vi "Alex Fails.vi"() -> ()   [LabVIEW 2014]
doc: "This VI is called when autonomous begins, and will automatically be terminated when autonomous ends. You can carry out timed or sensor driven robot movement independently without needing to return to the caller."
uses:
  Robot/Auto/Autonomous Modes.ctl
  Robot/Main/Elevator/Elevator States.ctl
  Robot/Main/Arms/Arm clapper state.ctl
  <vilib>/Rock Robotics/Network Tables/SD Read Number.vi
panel:
  in  "Forward Speed 2":dbl=0.8
  in  "Forward Speed":dbl=0.55 format="%#_13g"
  in  "Distance (in)":dbl=108.0
  in  "Turn Left Distance (m)":dbl=108.0 format="%#_13g"
  in  "Turn Left Speed":dbl=0.5
  in  "Turn Right Speed":dbl=0.5
  in  "Turn Right Distance (m)":dbl=108.0 format="%#_13g"
  in  "Move Speed":dbl=0.5 format="%#_13g"
  in  "Move Time (s)":dbl=2.5 format="%#_13g"
  # "THREE TOTE"
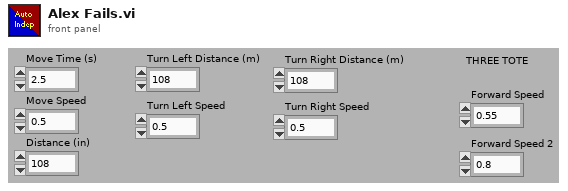
[diagram p1: front panel]
types:
  T1 = typedef "Autonomous Modes.ctl" = enum16{"3 Tote", "Turn Left, Drive to Auto", "Turn Right, Drive to Auto", "1 Bin", "Move To Auto Zone", "Do Nothing"}
  T2 = typedef "Auto Notifiers.ctl" = cluster{"Auto to Clap":refnum<notifier>, "Clap to Auto":refnum<notifier>, "Auto to Angle":refnum<notifier>, "Angle to Auto":refnum<notifier>, "Auto to Roller":refnum<notifier>, "Drive Distance Speed":refnum<notifier>, "Drive Distance Distance":refnum<notifier>, "Auto Done?":refnum<notifier>, "Keep Straight?":refnum<notifier>, "Turn 90?":refnum<notifier>}
  T3 = typedef "Auto Refs.ctl" = cluster{"Ultrasonic Forward":T4, "Ultrasonic Back":T4, "Strafe Motor":T8, "Drive Motors":T17, "Gyro":T18}
  T4 = typedef "WPI_SonarMB1010AnalogDeviceRef.ctl" = cluster{"AIDeviceRef":T5, "Scaling factor (V/in)":dbl, "Average Bits":u8}
  T5 = typedef "WPI_AnalogChannelDevRef.ctl" = cluster{"DevStatus":errorcluster, "Controller":T6, "Analog Channel":T7}
  T6 = typedef "FPGA_TypedefAnalogModule.ctl" = enum16{"Controller 1"}
  T7 = typedef "FPGA_AIChannel.ctl" = enum8{"AI 0", "AI 1", "AI 2", "AI 3", "AI MXP 0", "AI MXP 1", "AI MXP 2", "AI MXP 3", "Invalid"}
  T8 = typedef "WPI_MotorControlDeviceRef.ctl" = cluster{"DeviceStatus":errorcluster, "Type":T9, "PWM":cluster{"Controller":T10, "PWM Channel":T11, "DeadBand":T12}, "CAN":cluster{"Device Number":u8, "Control Mode":T13, "Semaphore":T14, "Max Vout":dbl, "TalonSRX Control Mode":T15}, "Invert":bool, "TransformRef":T16, "InvTransformRef":T16}
  T9 = typedef "WPI_MotorControlType.ctl" = enum16{"PWM", "CAN", "CANTalonSRX"}
  T10 = typedef "FPGA_TypedefDigitalModule.ctl" = enum16{"Controller 1"}
  T11 = typedef "FPGA_DIOPWMChannel.ctl" = enum8{"PWM 0", "PWM 1", "PWM 2", "PWM 3", "PWM 4", "PWM 5", "PWM 6", "PWM 7", "PWM 8", "PWM 9", "PWM MXP 0", "PWM MXP 1", "PWM MXP 2", "PWM MXP 3", "PWM MXP 4", "PWM MXP 5", "PWM MXP 6", "PWM MXP 7", "PWM MXP 8", "PWM MXP 9", "Invalid"}
  T12 = typedef "WPI_PWMDeadband.ctl" = cluster{"Name":string, "maxPositivePwm":i32, "minPositivePwm":i32, "centerPwm":i32, "maxNegativePwm":i32, "minNegativePwm":i32, "angularRange":u16}
  T13 = typedef "WPI_CANJaguar_ControlMode.ctl" = enum8{"Percent VBus", "Current", "Speed", "Position", "Voltage"}
  T14 = typedef "Semaphore RefNum" = refnum<k1>
  T15 = typedef "WPI_CANTalonSRX_APIControlMode.ctl" = enum8{"Percent VBus", "Speed", "Position", "Slave", "Unchanged / Invalid"}
  T16 = typedef "WPI_PWMTransform_ConPane.ctl" = refnum<vi>
  T17 = typedef "WPI_RobotDriveDevRef.ctl" = cluster{"DevStatus":errorcluster, "Motors[]":T8[], "Square Inputs":bool, "Max Output":dbl}
  T18 = typedef "WPI_GyroDevRef.ctl" = cluster{"DevStatus":errorcluster, "Analog Module":T6, "Analog Channel":T7, "Offset":dbl, "Gain (VoltsPerDegree/Second)":dbl}
  T19 = typedef "Arm clapper state.ctl" = enum16{"In", "Tote Closed", "Bin Closed", "Straight", "Open"}
  T20 = typedef "Elevator States.ctl" = enum16{"Ground", "Tote 1", "Tote 2", "Tote 3", "Tote 4", "Tote 5", "Tote 6"}
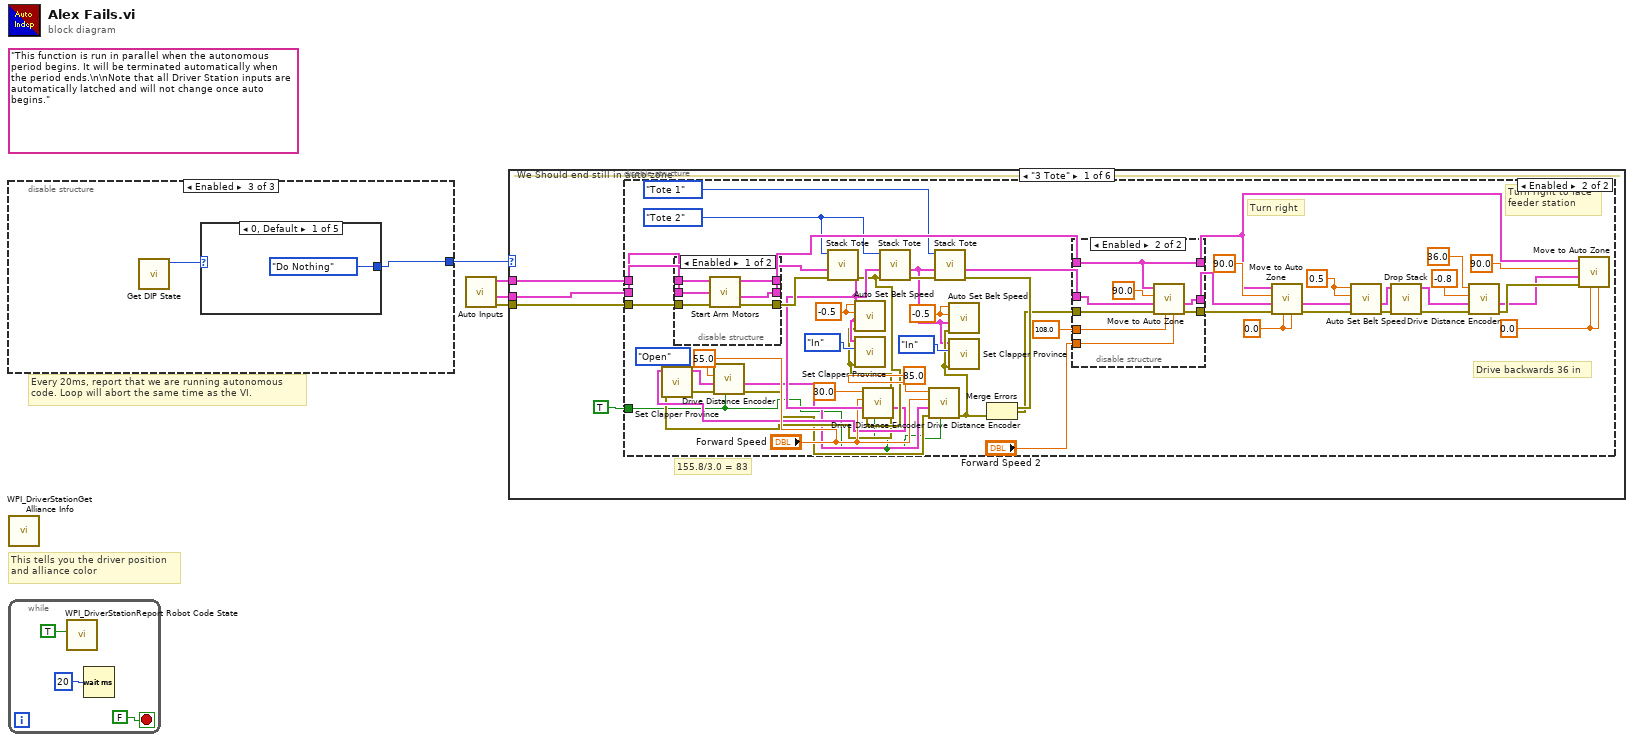
[diagram p0: block diagram]
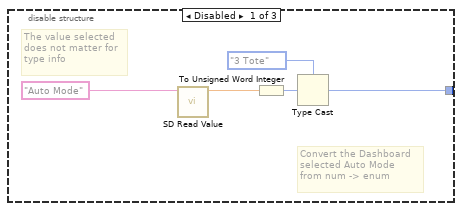
[diagram p2: hidden frame]
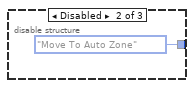
[diagram p3: hidden frame]
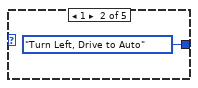
[diagram p4: hidden frame]
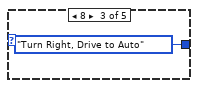
[diagram p5: hidden frame]
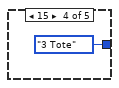
[diagram p6: hidden frame]
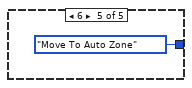
[diagram p7: hidden frame]
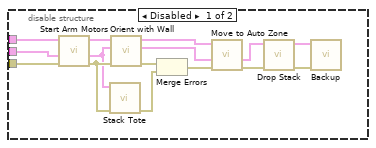
[diagram p8: hidden frame]
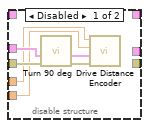
[diagram p10: hidden frame]
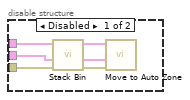
[diagram p12: hidden frame]
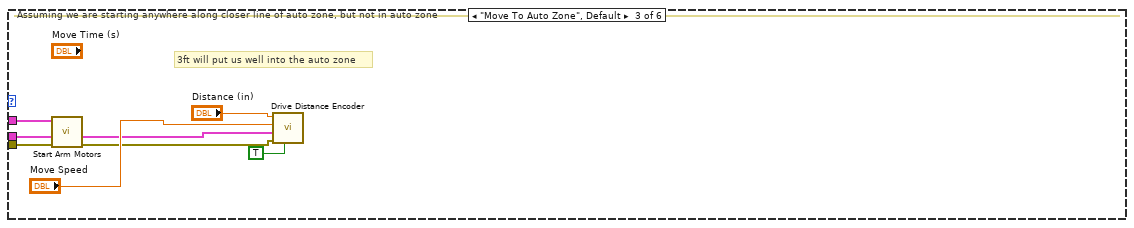
[diagram p13: hidden frame]
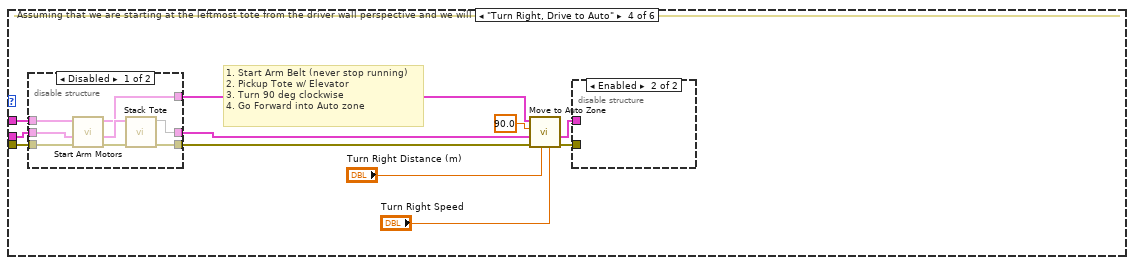
[diagram p14: hidden frame]
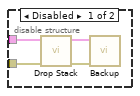
[diagram p15: hidden frame]
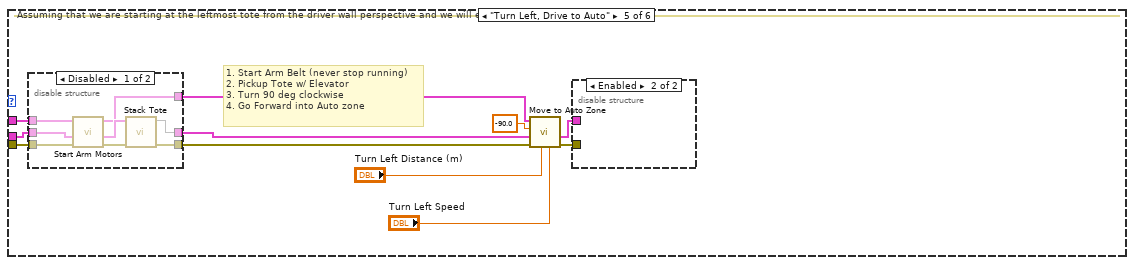
[diagram p17: hidden frame]
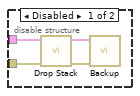
[diagram p18: hidden frame]
diagram:
  (unwired) "This function is run in parallel when the autonomous period begins. It will be terminated automatically when the period ends.\n\nNote that all Driver Station inputs are automatically latched and will not change once auto begins."
  # "Every 20ms, report that we are running autonomous\ncode. Loop will abort the same time as the VI."
  # "This tells you the driver position\nand alliance color"
  n1 = disable-structure shown="Enabled" {
    disable-tunnel: [w5 Autonomous_Modes."Move To Auto Zone" ("Auto Mode") w11] -> w1
    frame Disabled {
      # "The value selected\ndoes not matter for\ntype info"
      # "Convert the Dashboard\nselected Auto Mode\nfrom num -> enum"
      n2 = call-poly <vilib>:"SD Read Value.vi"("Name"="Auto Mode") -> ("Numeric"=w9:dbl)  [unwired: 8 in, 2 out]
      n3 = To Unsigned Word Integer(number=w9) -> (unsigned 16bit integer=w8:u16)
      n4 = Type Cast(type=Autonomous_Modes."3 Tote" ("Auto Mode"), x=w8) -> (*(type *) &x=w5:T1)
    }
    frame Disabled {
    }
    frame Enabled {
      n5 = call "Get DIP State.vi"() -> ("DIP State"=w12:u32)  [unwired: 10 in, 1 out]
      n6 = case shown="0, Default" w12 {
        tunnel: [Autonomous_Modes."Do Nothing" ("Auto Mode") Autonomous_Modes."Turn Left, Drive to Auto" ("Auto Mode") Autonomous_Modes."Turn Right, Drive to Auto" ("Auto Mode") Autonomous_Modes."3 Tote" ("Auto Mode") Autonomous_Modes."Move To Auto Zone" ("Auto Mode")] -> w11
        frame 0, Default {
        }
        frame 1 {
        }
        frame 8 {
        }
        frame 15 {
        }
        frame 6 {
        }
      }
    }
  }
  n7 = call <vilib>:"WPI_DriverStationGet Alliance Info.vi"() -> ()  [unwired: 12 out]
  n8 = while {
    stop <- FALSE stop-if-true
    n9 = call <vilib>:"WPI_DriverStationReport Robot Code State.vi"("Autonomous"=TRUE) -> ()  [unwired: 10 in, 1 out]
    n10 = Wait (ms)(milliseconds to wait=u32 20) -> ()  [unwired: 1 out]
  }
  n11 = call "Auto Inputs.vi"() -> ("error out"=w2:errorcluster, "Auto Notifiers Out"=w3:T2, "Auto Refs"=w4:T3)  [unwired: 9 in]
  n12 = case shown="\"3 Tote\"" w1 {
    tunnel: w4 -> [w22 w117 w126 w136 w162 _]
    tunnel: w3 -> [w24 w116 w128 w140 w166 _]
    tunnel: w2 -> [w23 w115 w130 w139 w165 _]
    frame "3 Tote" {
      # "155.8/3.0 = 83"
      # "We Should end still in auto zone"
      n13 = disable-structure shown="Enabled" {
        disable-tunnel: w24 -> [w32 w90]
        disable-tunnel: w23 -> [w31 w91]
        disable-tunnel: w22 -> [w25 w89]
        disable-tunnel: TRUE -> [_ w40]
        frame Disabled {
          n14 = call "Start Arm Motors.vi"("error in"=w31, "Auto Notifiers In"=w32, "Auto Refs"=w25) -> ("error out"=w37:errorcluster, "Auto Notifiers Out"=w34:T2, "Auto Refs"=w36:T3)  [unwired: 6 in]
          n15 = call "Stack Tote.vi"("error in"=w37, "End at"=w34) -> ("error out"=w38:errorcluster)  [unwired: 8 in, 1 out]
          n16 = call "Orient with Wall.vi"("error in"=w37, "Auto Notifiers In"=w34, "Auto Refs"=w36) -> ("error out"=w35:errorcluster, "Auto Notifiers Out"=w33:T2, "Auto Refs"=w26:T3)  [unwired: 6 in]
          n17 = Merge Errors(w35, w38) -> (w39:errorcluster)
          n18 = call "Move to Auto Zone.vi"("error in"=w39, "Auto Notifiers In"=w33, "Auto Refs"=w26) -> ("error out"=w29:errorcluster, "Auto Notifiers Out"=w28:T2)  [unwired: 7 in]
          n19 = call "Drop Stack.vi"("error in"=w29, "Auto Notifiers In"=w28) -> ("error out"=w30:errorcluster, "Auto Notifiers Out"=w27:T2)  [unwired: 8 in]
          n20 = call "Backup.vi"("error in"=w30, "Auto Notifiers In"=w27) -> ()  [unwired: 8 in, 2 out]
        }
        frame Enabled {
          w56 = -0.5 ("Right Belt")
          w57 = -0.5 ("Right Belt")
          w73 = Elevator_States."Tote 2" ("New State")
          w81 = 0.0 ("Distance (m)")
          w82 = 0.0 ("Distance (m)")
          w61 = 0.5
          # "Drive backwards 36 in"
          # "Turn right to face\nfeeder station"
          # "Turn right"
          n21 = disable-structure shown="Enabled" {
            disable-tunnel: w91 -> [w97 w98]
            disable-tunnel: w90 -> [w96 w100]
            disable-tunnel: w89 -> [w95 w99]
            disable-tunnel: [w94 w98] -> w77
            disable-tunnel: [w93 w100] -> w78
            disable-tunnel: [w92 w99] -> w86
            frame Enabled {
              n22 = call "Start Arm Motors.vi"("error in"=w97, "Auto Notifiers In"=w96, "Auto Refs"=w95) -> ("error out"=w94:errorcluster, "Auto Notifiers Out"=w93:T2, "Auto Refs"=w92:T3)  [unwired: 6 in]
            }
            frame Disabled {
            }
          }
          n23 = call "Stack Tote.vi"("error in"=w77, "Auto Notifiers In"=w78, "End at"=w73) -> ("error out"=w51:errorcluster, "Auto Notifiers Out"=w52:T2)  [unwired: 7 in]
          n24 = call "Drive Distance Encoder.vi"("Gyro Sync?"=w40, "error in"=w51, "Auto Notifiers In"=w52, "Speed"="Forward Speed", "Distance (in)"=30.0) -> ("error out"=w43:errorcluster, "Auto Notifiers Out"=w44:T2)  [unwired: 5 in]
          n25 = call "Set Clapper Province.vi"("error in"=w43, "Enum"=Arm_clapper_state."Open", "Auto Notifiers In"=w44) -> ("error out"=w47:errorcluster, "Auto Notifiers Out"=w48:T2)  [unwired: 7 in]
          n26 = call "Drive Distance Encoder.vi"("Gyro Sync?"=w40, "error in"=w47, "Auto Notifiers In"=w48, "Speed"="Forward Speed", "Distance (in)"=55.0) -> ("error out"=w42:errorcluster, "Auto Notifiers Out"=w41:T2)  [unwired: 5 in]
          n27 = call "Auto Set Belt Speed.vi"("error in"=w43, "Auto Notifiers In"=w52, "Right Belt"=w57, "Left Belt"=w57) -> ()  [unwired: 6 in, 2 out]
          n28 = call "Set Clapper Province.vi"("error in"=w43, "Enum"=Arm_clapper_state."In", "Auto Notifiers In"=w52) -> ()  [unwired: 7 in, 2 out]
          n29 = call "Stack Tote.vi"("error in"=w51, "Auto Notifiers In"=w52, "End at"=w73) -> ("error out"=w76:errorcluster, "Auto Notifiers Out"=w53:T2)  [unwired: 7 in]
          n30 = call "Drive Distance Encoder.vi"("Gyro Sync?"=w40, "error in"=w42, "Auto Notifiers In"=w41, "Speed"="Forward Speed", "Distance (in)"=85.0) -> ("error out"=w54:errorcluster)  [unwired: 5 in, 1 out]
          n31 = call "Stack Tote.vi"("error in"=w76, "Auto Notifiers In"=w53, "End at"=Elevator_States."Tote 1" ("New State")) -> ("error out"=w75:errorcluster, "Auto Notifiers Out"=w88:T2)  [unwired: 7 in]
          n32 = call "Auto Set Belt Speed.vi"("error in"=w54, "Auto Notifiers In"=w53, "Right Belt"=w56, "Left Belt"=w56) -> ()  [unwired: 6 in, 2 out]
          n33 = call "Set Clapper Province.vi"("error in"=w54, "Enum"=Arm_clapper_state."In", "Auto Notifiers In"=w53) -> ()  [unwired: 7 in, 2 out]
          n34 = Merge Errors(w75, w54) -> (w74:errorcluster)
          n35 = disable-structure shown="Enabled" {
            disable-tunnel: w74 -> [w106 w114]
            disable-tunnel: w88 -> [w105 w113]
            disable-tunnel: "Forward Speed 2" -> [w102 w110]
            disable-tunnel: 108.0 ("Distance (in)") -> [w101 w111]
            disable-tunnel: w86 -> [_ w107]
            disable-tunnel: [_ w109] -> w85
            disable-tunnel: [_ w108] -> w84
            disable-tunnel: [_ w107] -> w79
            frame Disabled {
              n36 = call "Turn 90 deg.vi"("error in"=w106, "Auto Notifiers In"=w105) -> ("error out"=w104:errorcluster, "Auto Notifiers Out"=w103:T2)  [unwired: 8 in]
              n37 = call "Drive Distance Encoder.vi"("error in"=w104, "Auto Notifiers In"=w103, "Speed"=w102, "Distance (in)"=w101) -> ()  [unwired: 6 in, 2 out]
            }
            frame Enabled {
              n38 = call "Move to Auto Zone.vi"("Speed"=w110, "Distance (m)"=w111, "error in"=w114, "Auto Notifiers In"=w113, "Rotation (deg)"=90.0, "Auto Refs"=w107) -> ("error out"=w109:errorcluster, "Auto Notifiers Out"=w108:T2)  [unwired: 4 in]
            }
          }
          n39 = call "Move to Auto Zone.vi"("Speed"=w82, "Distance (m)"=w82, "error in"=w85, "Auto Notifiers In"=w84, "Rotation (deg)"=90.0, "Auto Refs"=w79) -> ("error out"=w63:errorcluster, "Auto Notifiers Out"=w62:T2)  [unwired: 4 in]
          n40 = call "Auto Set Belt Speed.vi"("error in"=w63, "Auto Notifiers In"=w62, "Right Belt"=w61, "Left Belt"=w61) -> ("error out"=w65:errorcluster, "Auto Notifiers Out"=w64:T2)  [unwired: 6 in]
          n41 = call "Drop Stack.vi"("error in"=w65, "Auto Notifiers In"=w64) -> ("error out"=w67:errorcluster, "Auto Notifiers Out"=w66:T2)  [unwired: 8 in]
          n42 = call "Drive Distance Encoder.vi"("error in"=w67, "Auto Notifiers In"=w66, "Speed"=-0.8, "Distance (in)"=36.0) -> ("error out"=w69:errorcluster, "Auto Notifiers Out"=w68:T2)  [unwired: 6 in]
          n43 = call "Move to Auto Zone.vi"("Speed"=w81, "Distance (m)"=w81, "error in"=w69, "Auto Notifiers In"=w68, "Rotation (deg)"=90.0 ("Distance (in)"), "Auto Refs"=w79) -> ()  [unwired: 4 in, 2 out]
        }
      }
    }
    frame "1 Bin" {
      # "1. Pick Up Bin w/ Elevator\n2. Turn 90 deg counterclockwise\n3. Go forward into auto zone\n4. DO NOT drop bin"
      # "Assuming we are starting on top of the leftmost bin from the driver wall perspective and we will end in auto zone"
      n44 = disable-structure shown="Enabled" {
        disable-tunnel: w117 -> [w121 _]
        disable-tunnel: w116 -> [w120 _]
        disable-tunnel: w115 -> [w118 _]
        frame Disabled {
          n45 = call "Stack Bin.vi"("error in"=w118, "Auto Notifiers In"=w120, "Auto Refs"=w121) -> ("error out"=w123:errorcluster, "Auto Notifiers Out"=w119:T2, "Auto Refs"=w122:T3)  [unwired: 6 in]
          n46 = call "Move to Auto Zone.vi"("error in"=w123, "Auto Notifiers In"=w119, "Auto Refs"=w122) -> ()  [unwired: 7 in, 2 out]
        }
        frame Enabled {
        }
      }
    }
    frame "Move To Auto Zone", Default {
      # "3ft will put us well into the auto zone"
      # "Assuming we are starting anywhere along closer line of auto zone, but not in auto zone"
      n47 = call "Start Arm Motors.vi"("error in"=w130, "Auto Notifiers In"=w128, "Auto Refs"=w126) -> ("error out"=w129:errorcluster, "Auto Notifiers Out"=w127:T2)  [unwired: 6 in, 1 out]
      n48 = call "Drive Distance Encoder.vi"("Gyro Sync?"=TRUE, "error in"=w129, "Auto Notifiers In"=w127, "Speed"="Move Speed", "Distance (in)"="Distance (in)") -> ()  [unwired: 5 in, 2 out]
    }
    frame "Turn Right, Drive to Auto" {
      # "1. Start Arm Belt (never stop running)\n2. Pickup Tote w/ Elevator\n3. Turn 90 deg clockwise\n4. Go Forward into Auto zone"
      # "Assuming that we are starting at the leftmost tote from the driver wall perspective and we will end in auto zone"
      n49 = disable-structure shown="Disabled" {
        disable-tunnel: [w154 w155] -> w141
        disable-tunnel: w140 -> [w152 w156]
        disable-tunnel: w139 -> [w151 w155]
        disable-tunnel: [w149 w156] -> w138
        disable-tunnel: w136 -> [w148 w157]
        disable-tunnel: [w147 w157] -> w135
        frame Disabled {
          n50 = call "Start Arm Motors.vi"("error in"=w151, "Auto Notifiers In"=w152, "Auto Refs"=w148) -> ("error out"=w153:errorcluster, "Auto Notifiers Out"=w150:T2, "Auto Refs"=w147:T3)  [unwired: 6 in]
          n51 = call "Stack Tote.vi"("error in"=w153, "End at"=w150) -> ("error out"=w154:errorcluster, 3:w149)  [unwired: 7 in, 1 out]
        }
        frame Enabled {
        }
      }
      n52 = call "Move to Auto Zone.vi"("Speed"="Turn Right Speed", "Distance (m)"="Turn Right Distance (m)", "error in"=w141, "Auto Notifiers In"=w138, "Rotation (deg)"=90.0, "Auto Refs"=w135) -> ("error out"=w142:errorcluster, "Auto Notifiers Out"=w137:T2)  [unwired: 4 in]
      n53 = disable-structure shown="Enabled" {
        disable-tunnel: w142 -> [w145 _]
        disable-tunnel: w137 -> [w144 _]
        frame Disabled {
          n54 = call "Drop Stack.vi"("error in"=w145, "Auto Notifiers In"=w144) -> ("error out"=w146:errorcluster, "Auto Notifiers Out"=w143:T2)  [unwired: 8 in]
          n55 = call "Backup.vi"("error in"=w146, "Auto Notifiers In"=w143) -> ()  [unwired: 8 in, 2 out]
        }
        frame Enabled {
        }
      }
    }
    frame "Turn Left, Drive to Auto" {
      # "1. Start Arm Belt (never stop running)\n2. Pickup Tote w/ Elevator\n3. Turn 90 deg clockwise\n4. Go Forward into Auto zone"
      # "Assuming that we are starting at the leftmost tote from the driver wall perspective and we will end in auto zone"
      n56 = disable-structure shown="Disabled" {
        disable-tunnel: [w180 w181] -> w167
        disable-tunnel: w166 -> [w178 w182]
        disable-tunnel: w165 -> [w177 w181]
        disable-tunnel: [w175 w182] -> w164
        disable-tunnel: w162 -> [w174 w183]
        disable-tunnel: [w173 w183] -> w161
        frame Disabled {
          n57 = call "Start Arm Motors.vi"("error in"=w177, "Auto Notifiers In"=w178, "Auto Refs"=w174) -> ("error out"=w179:errorcluster, "Auto Notifiers Out"=w176:T2, "Auto Refs"=w173:T3)  [unwired: 6 in]
          n58 = call "Stack Tote.vi"("error in"=w179, "End at"=w176) -> ("error out"=w180:errorcluster, 3:w175)  [unwired: 7 in, 1 out]
        }
        frame Enabled {
        }
      }
      n59 = call "Move to Auto Zone.vi"("Speed"="Turn Left Speed", "Distance (m)"="Turn Left Distance (m)", "error in"=w167, "Auto Notifiers In"=w164, "Rotation (deg)"=-90.0, "Auto Refs"=w161) -> ("error out"=w168:errorcluster, "Auto Notifiers Out"=w163:T2)  [unwired: 4 in]
      n60 = disable-structure shown="Enabled" {
        disable-tunnel: w168 -> [w171 _]
        disable-tunnel: w163 -> [w170 _]
        frame Disabled {
          n61 = call "Drop Stack.vi"("error in"=w171, "Auto Notifiers In"=w170) -> ("error out"=w172:errorcluster, "Auto Notifiers Out"=w169:T2)  [unwired: 8 in]
          n62 = call "Backup.vi"("error in"=w172, "Auto Notifiers In"=w169) -> ()  [unwired: 8 in, 2 out]
        }
        frame Enabled {
        }
      }
    }
    frame "Do Nothing" {
    }
  }
